vi "AlliGator Get Series Dataset Type.vi"(8 "Error In":errorcluster, 11 "AlliGator Dataset Series Type":T2) -> (0 "Error Out":errorcluster, 3 "FLI Dataset Type":T1)   [LabVIEW 2021, in "AlliGator Scripts.lvlib"]
doc: "Converts Dataset Series type to FLI Dataset type enum."
uses:
  AlliGator Scripts.lvlib
  Files/AlliGator Data Series Type.ctl
  Files/AlliGator FLI Dataset Type.ctl
  Files/AlliGator Files.lvlib
panel:
  # "see the AlliGator License on the block diagram (Ctrl+E or Window:Show Block Diagram)"
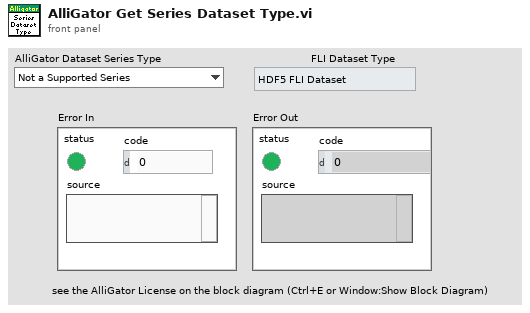
[diagram p1: front panel]
types:
  T1 = typedef "AlliGator Files.lvlib/AlliGator FLI Dataset Type.ctl" = enum16{"HDF5 FLI Dataset", "Gate Image Folder", ".sdt FLI Dataset (Becker & Hickl)", ".ptu FLI Dataset (PicoQuant)", "SS1 FLI Dataset", "SS2 FLI Dataset", "I/m/phi Dataset", ".bin FLI Dataset (PicoQuant Binned)", ".bin FLI Dataset (Piccolo Binned)"}
  T2 = typedef "AlliGator Files.lvlib/AlliGator Data Series Type.ctl" = enum16{"Not a Supported Series", "Gate Images Folder Series", "SwissSPAD 2 Dataset Series", "B&H FLI Dataset Series", "PicoQuant PTU FLI Dataset Series", "PicoQuant BIN FLI Dataset Series", "Piccolo hist BIN FLI Dataset Series", "HDF5 FLI Dataset Series"}
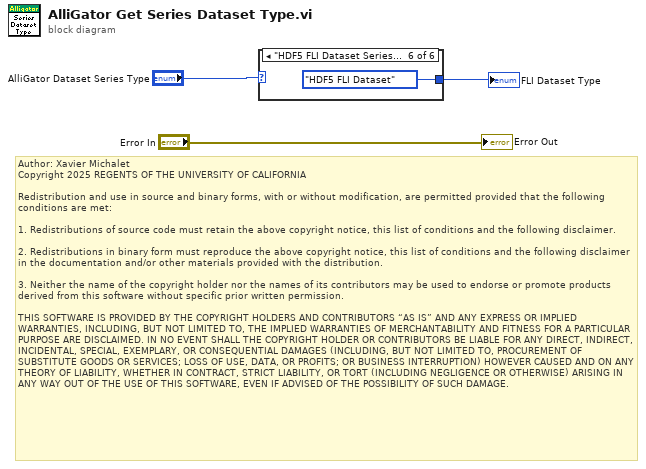
[diagram p0: block diagram]
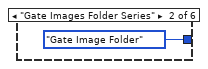
[diagram p3: hidden frame]
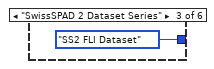
[diagram p4: hidden frame]
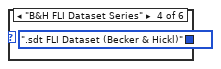
[diagram p5: hidden frame]
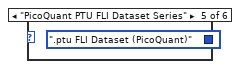
[diagram p6: hidden frame]
diagram:
  # "Author: Xavier Michalet\nCopyright 2025 REGENTS OF THE UNIVERSITY OF CALIFORNIA\n\nRedistribution and use in source and binary forms, with or without modification, are permitted provided that the following conditions are met:\n\n1. Redistributions of source code must retain the above copyright notice, this list of conditions and the following disclaimer.\n\n2. Redistributions in binary form must reproduce the above copyright notice, this list of conditions and the following disclaimer in the documentation and/or other materials provided with the distribution.\n\n3. Neither the name of the copyright holder nor the names of its contributors may be used to endorse or promote products derived from this software without specific prior written permission.\n\nTHIS SOFTWARE IS PROVIDED BY THE COPYRIGHT HOLDERS AND CONTRIBUTORS “AS IS” AND ANY EXPRESS OR IMPLIED WARRANTIES, INCLUDING, BUT NOT LIMITED TO, THE IMPLIED WARRANTIES OF MERCHANTABILITY AND FITNESS FOR A PARTICULAR PURPOSE ARE DISCLAIMED. IN NO EVENT SHALL THE COPYRIGHT HOLDER OR CONTRIBUTORS BE LIABLE FOR ANY DIRECT, INDIRECT, INCIDENTAL, SPECIAL, EXEMPLARY, OR CONSEQUENTIAL DAMAGES (INCLUDING, BUT NOT LIMITED TO, PROCUREMENT OF SUBSTITUTE GOODS OR SERVICES; LOSS OF USE, DATA, OR PROFITS; OR BUSINESS INTERRUPTION) HOWEVER CAUSED AND ON ANY THEORY OF LIABILITY, WHETHER IN CONTRACT, STRICT LIABILITY, OR TORT (INCLUDING NEGLIGENCE OR OTHERWISE) ARISING IN ANY WAY OUT OF THE USE OF THIS SOFTWARE, EVEN IF ADVISED OF THE POSSIBILITY OF SUCH DAMAGE."
  n1 = case shown="\"HDF5 FLI Dataset Series\"" "AlliGator Dataset Series Type" {
    tunnel: [_ AlliGator_FLI_Dataset_Type."Gate Image Folder" ("FLI Dataset Type") AlliGator_FLI_Dataset_Type."SS2 FLI Dataset" ("FLI Dataset Type") AlliGator_FLI_Dataset_Type.".sdt FLI Dataset (Becker & Hickl)" ("FLI Dataset Type") AlliGator_FLI_Dataset_Type.".ptu FLI Dataset (PicoQuant)" ("FLI Dataset Type") AlliGator_FLI_Dataset_Type."HDF5 FLI Dataset" ("FLI Dataset Type")] -> w2
    frame "Not a Supported Series", Default {
    }
    frame "Gate Images Folder Series" {
    }
    frame "SwissSPAD 2 Dataset Series" {
    }
    frame "B&H FLI Dataset Series" {
    }
    frame "PicoQuant PTU FLI Dataset Series" {
    }
    frame "HDF5 FLI Dataset Series" {
    }
  }
  "FLI Dataset Type" <- w2
  "Error Out" <- "Error In"
